vi "encoder task.vi"(11 "AIDeviceRef":T1) -> ()   [LabVIEW 2011]
uses:
  <vilib>/Rock Robotics/WPI/AnalogChannel/WPI_AnalogChannelDevRef.ctl
  <vilib>/Rock Robotics/SystemInterfaces/Typedef/FPGA_TypedefAnalogModule.ctl
  <vilib>/Rock Robotics/SystemInterfaces/AI/FPGA_AIChannel.ctl
  Robot Global Data.vi
panel:
  out "Turn count":dbl
  out "Above Threshold":bool
  in  "Threshold":dbl(slide)=3.0232558139534884 scale=0.0..5.0
  out "Waveform Chart":dbl(graph)
  out "Voltage":dbl
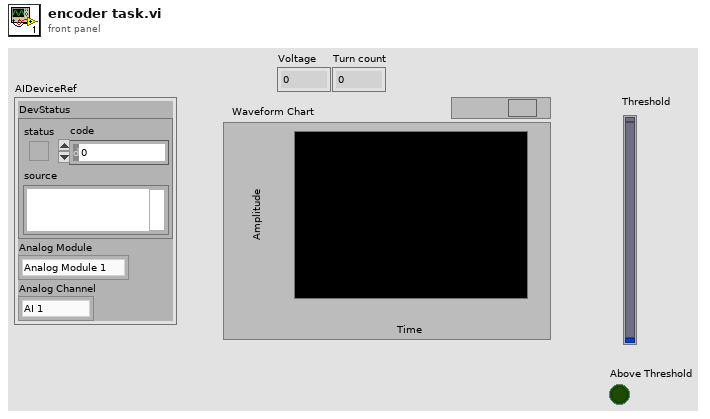
[diagram p1: front panel]
types:
  T1 = typedef "WPI_AnalogChannelDevRef.ctl" = cluster{"DevStatus":errorcluster, "Analog Module":T2, "Analog Channel":T3}
  T2 = typedef "FPGA_TypedefAnalogModule.ctl" = enum16{"Analog Module 1", "Analog Module 2"}
  T3 = typedef "FPGA_AIChannel.ctl" = enum8{"AI 1", "AI 2", "AI 3", "AI 4", "AI 5", "AI 6", "AI 7", "AI 8", "Invalid"}
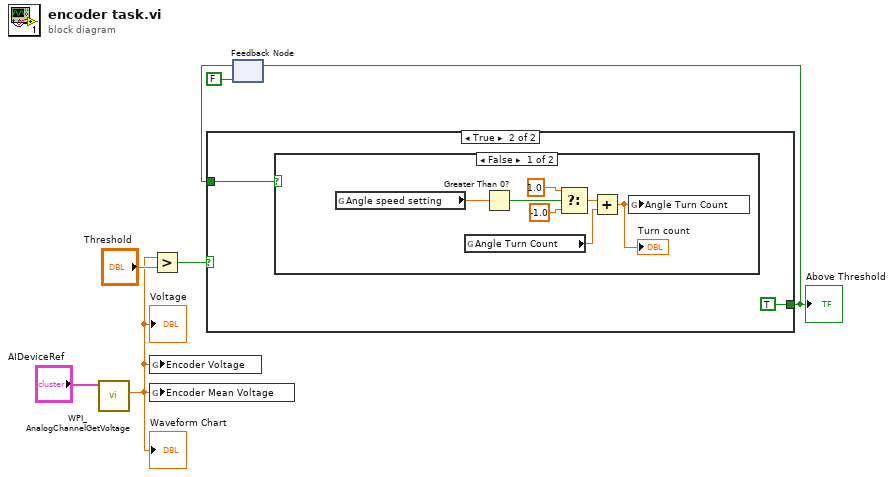
[diagram p0: block diagram]
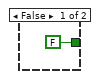
[diagram p2: hidden frame]
diagram:
  n1 = call <vilib>:"WPI_AnalogChannelGetVoltage.vi"("AIDeviceRef"="AIDeviceRef") -> ("Voltage"=w5:dbl)  [unwired: 8 in, 2 out]
  "Voltage" <- w5
  "Waveform Chart" <- w5
  n2 = global write "Robot Global Data.vi" "Encoder Voltage"(w5) -> ()
  n3 = global write "Robot Global Data.vi" "Encoder Mean Voltage"(w5) -> ()
  n4 = Greater?(x=w5, y="Threshold") -> (0:w4:bool)
  n5 = feedback #1(FALSE) -> (w3:bool)
  n6 = case shown="True" w4 {
    tunnel: w3 -> [_ w9]
    tunnel: [FALSE TRUE] -> w1
    frame False {
    }
    frame True {
      n7 = case shown="False" w9 {
        frame False {
          n8 = global read "Robot Global Data.vi" "Angle speed setting"() -> (w17:dbl)
          n9 = global read "Robot Global Data.vi" "Angle Turn Count"() -> (w13:dbl)
          n10 = Greater Than 0?(x=w17) -> (x > 0?=w16:bool)
          n11 = Select(t=1.0, s=w16, f=-1.0) -> (s? t:f=w12:dbl)
          n12 = Add(x=w12, y=w13) -> (x+y=w11:dbl)
          "Turn count" <- w11
          n13 = global write "Robot Global Data.vi" "Angle Turn Count"(w11) -> ()
        }
        frame True {
          # "Dont increment turn count as we only\ncount threshold crossings"
        }
      }
    }
  }
  "Above Threshold" <- w1
  n14 = feedback-in #1(w1) -> ()
